vi "Convert radians per sec to rpm.vi"(11 "speed in":dbl[unit]) -> (3 "speed out (rpm)":dbl)   [LabVIEW 2019]
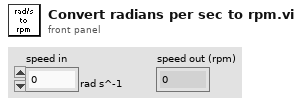
[diagram p1: front panel]
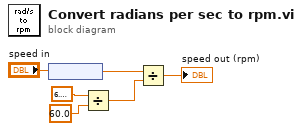
[diagram p0: block diagram]
diagram:
  n1 = node("speed in") -> (w6:dbl)
  n2 = Divide(x=6.283185307179586, y=60.0) -> (x/y=w3:dbl)
  n3 = Divide(x=w6, y=w3) -> (x/y=→"speed out (rpm)":dbl)
